vi "Open System Definition.vi"(8 "error in (no error)":errorcluster, 11 "System Definition File":path) -> (0 "error out":errorcluster, 1 "targets refnums":refnum<k24>[](array[refnum]), 2 "root refnum":refnum<k24>, 3 "system definition refnum":refnum<k24>)   [LabVIEW 2018, in "Bitfile Reload System Tests.lvclass"]
uses:
  Bitfile Reload System Tests.lvclass
  NationalInstruments.VeriStand.SystemDefinitionAPI
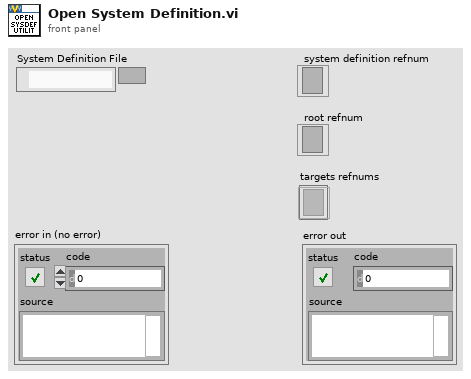
[diagram p1: front panel]
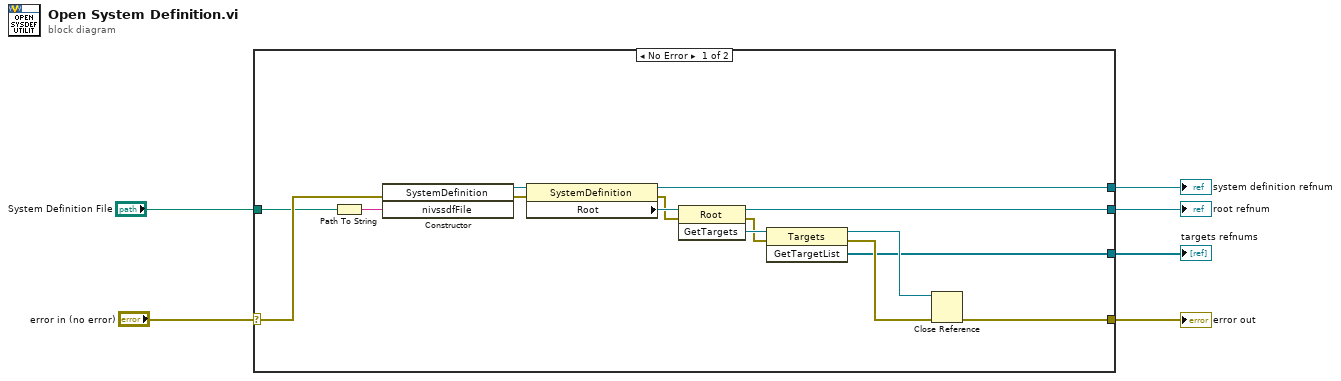
[diagram p0: block diagram]
diagram:
  n1 = case shown="No Error" "error in (no error)" {
    selector: "error in (no error)" -> [w14 w22]
    tunnel: [w13 w22] -> w5
    tunnel: "System Definition File" -> [w12 _]
    tunnel: [w11 _] -> w3
    tunnel: [w10 _] -> w2
    tunnel: [w7 _] -> w1
    frame No Error {
      n2 = Path To String(path=w12) -> (string=w15:string)
      n3 = constructor class="SystemDefinition"(error in=w14, "nivssdfFile"=w15) -> (reference out=w17:refnum<k24>, error out=w16:errorcluster)  [unwired: 2 in, 2 out]
      n4 = property class="SystemDefinition"(reference=w17, error in=w16) -> (reference out=w11:refnum<k24>, error out=w18:errorcluster, "Root"=w19:refnum<k24>)
      n5 = invoke class="Root" method="GetTargets"(reference=w19, error in=w18) -> (reference out=w10:refnum<k24>, error out=w20:errorcluster, "GetTargets"=w21:refnum<k24>)  [unwired: 1 in]
      n6 = invoke class="Targets" method="GetTargetList"(reference=w21, error in=w20) -> (reference out=w8:refnum<k24>, error out=w9:errorcluster, "GetTargetList"=w7:refnum<k24>[])  [unwired: 1 in]
      n7 = Close Reference(reference=w8, error in (no error)=w9) -> (error out=w13:errorcluster)
    }
    frame Error {
    }
  }
  "error out" <- w5
  "root refnum" <- w2
  "system definition refnum" <- w3
  "targets refnums" <- w1
